vi "Returns 1st and 2nd Display Value.vi"(8 "error in":errorcluster, 10 "Sets to Display":u16(ring) items=["1st Display", "2nd Display", "1st & 2nd Display"], 11 "VISA resource name":refnum<visa-resource-name>) -> (0 "error out":errorcluster, 2 "Return the Value":string, 3 "VISA resource name out":refnum<visa-resource-name>)   [LabVIEW 2021, in "DMM4.lvlib"]
uses:
  DMM4.lvlib
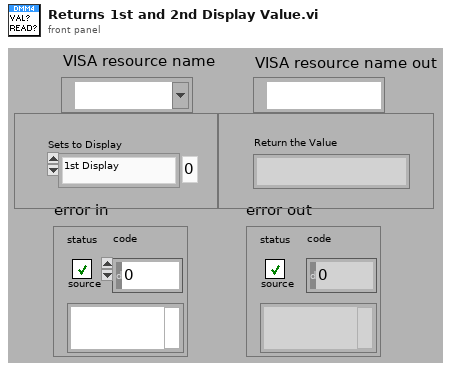
[diagram p1: front panel]
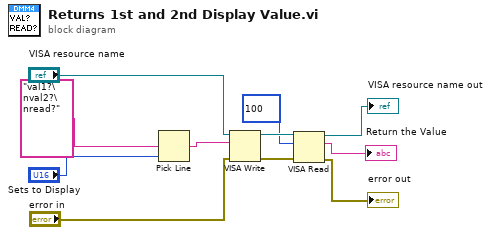
[diagram p0: block diagram]
diagram:
  n1 = Pick Line(multi-line string="val1?\nval2?\nread?", line index="Sets to Display") -> (output string=w7:string)  [unwired: 1 in]
  n2 = VISA Write(VISA resource name="VISA resource name", write buffer=w7, error in (no error)="error in") -> (VISA resource name out=w6:refnum<visa-resource-name>, error out=w5:errorcluster)  [unwired: 1 out]
  n3 = VISA Read(VISA resource name=w6, byte count=u32 100, error in (no error)=w5) -> (VISA resource name out=→"VISA resource name out":refnum<visa-resource-name>, read buffer=→"Return the Value":string, error out=→"error out":errorcluster)  [unwired: 1 out]
